vi "CALC_Phi_theta_etc_(offline).vi"(0 "Input cluster of data":T1, 1 "SB size":u8, 2 "Bridge swap":bool, 3 "Use alternative magnets orientation":bool, 4 "Twisted neck":bool) -> (5 "Animal coordinates":T2)   [LabVIEW 2018, in "Tracker.lvlib"]
uses:
  Tracker.lvlib
  Controls/CTL_Animal_Coordinates_and_Speed.ctl
  Controls/CTL_Cage_Coords.ctl
  Common_Resources.lvlib
  <vilib>/ptbypt/NI_PtbyPt.lvlib
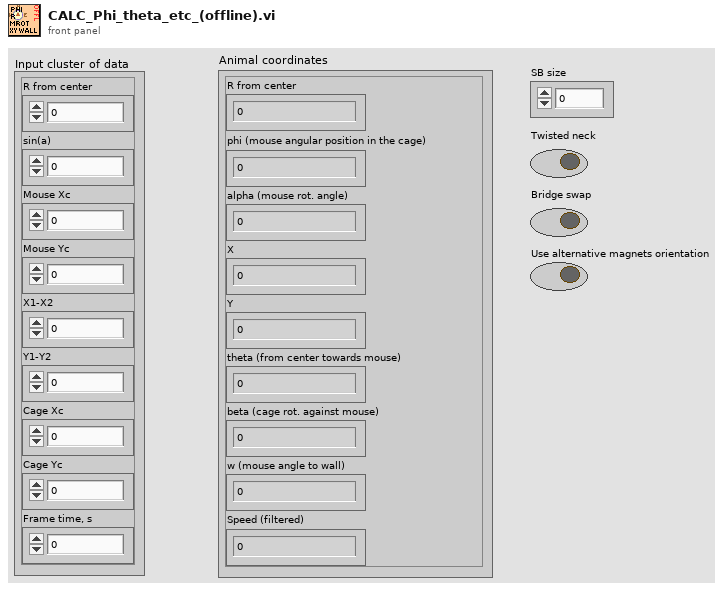
[diagram p1: front panel]
types:
  T1 = typedef "Common_Resources.lvlib/CTL_Cage_Coords.ctl" = cluster{"R from center":dbl, "sin(a)":dbl, "Mouse Xc":dbl, "Mouse Yc":dbl, "X1-X2":dbl, "Y1-Y2":dbl, "Cage Xc":dbl, "Cage Yc":dbl, "Frame time, s":dbl}
  T2 = typedef "Common_Resources.lvlib/CTL_Animal_Coordinates_and_Speed.ctl" = cluster{"R from center":dbl, "phi (mouse angular position in the cage)":dbl, "alpha (mouse rot. angle)":dbl, "X":dbl, "Y":dbl, "theta (from center towards mouse)":dbl, "beta (cage rot. against mouse)":dbl, "w (mouse angle to wall)":dbl, "Speed (filtered)":dbl}
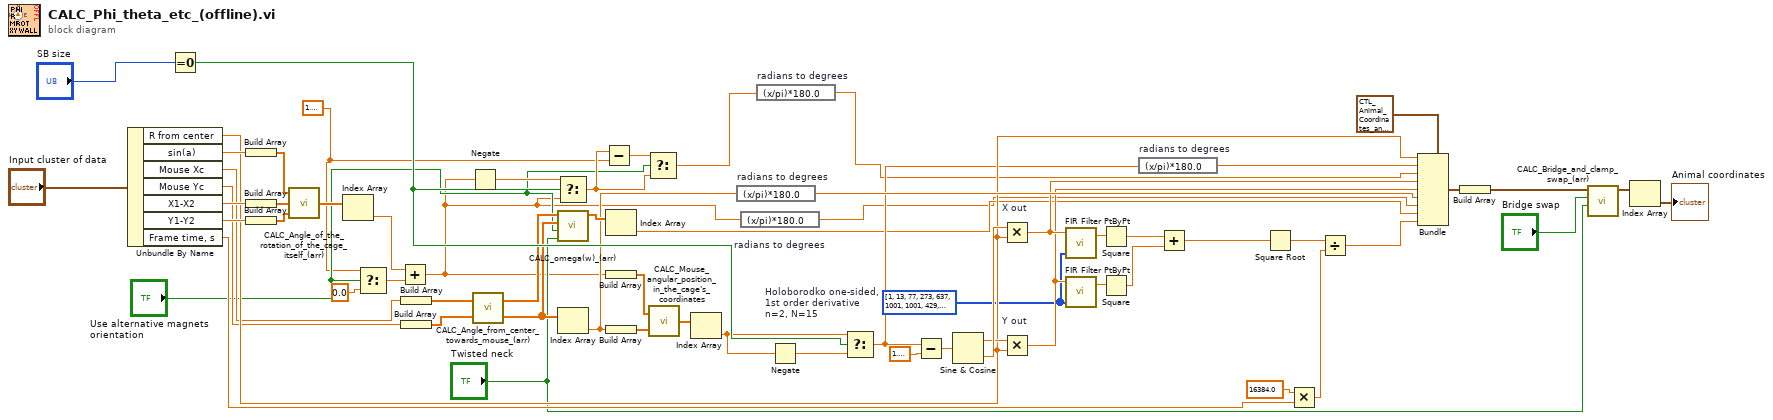
[diagram p0: block diagram]
diagram:
  w5 = 1.5707963267948966
  w36 = i32[] [1, 13, 77, 273, 637, 1001, 1001, 429, -429, -1001, -1001, -637, -273, -77, -13, -1]  # Holoborodko one-sided, 1st order derivative n=2, N=15
  n1 = Unbundle By Name("Input cluster of data") -> ("R from center"=w55:dbl, "sin(a)"=w58:dbl, "Mouse Xc"=w21:dbl, "Mouse Yc"=w20:dbl, "X1-X2"=w57:dbl, "Y1-Y2"=w56:dbl, "Frame time, s"=w30:dbl)
  n2 = Equal To 0?(x="SB size") -> (x = 0?=w39:bool)
  n3 = Build Array(w58) -> (w25:dbl[])
  n4 = Build Array(w57) -> (w24:dbl[])
  n5 = Build Array(w56) -> (w23:dbl[])
  n6 = call "CALC_Angle_of_the_rotation_of_the_cage_itself_(arr).vi"("Y1-Y2"=w23, "X1-X2"=w24, "sin(a)"=w25) -> ("Cage rot. angle, rad"=w50:dbl[])
  n7 = Index Array(array=w50) -> (element=w22:dbl)  [unwired: 1 in]
  n8 = Select(t=w5, s="Use alternative magnets orientation", f=0.0) -> (s? t:f=w48:dbl)
  n9 = Add(x=w22, y=w48) -> (x+y=w4:dbl)
  n10 = Build Array(w21) -> (w19:dbl[])
  n11 = Build Array(w20) -> (w18:dbl[])
  n12 = Negate(x=w4) -> (-x=w46:dbl)
  n13 = call "CALC_Angle_from_center_towards_mouse_(arr).vi"("Mouse Yc"=w18, "Mouse Xc"=w19) -> ("abs(theta) < pi, rad"=w11:dbl[], "theta, rad"=w12:dbl[])
  n14 = Select(t=w46, s=w39, f=w4) -> (s? t:f=w47:dbl)
  n15 = call "CALC_omega(w)_(arr).vi"("Twisted neck (F)"="Twisted neck", "Alt. magnets orientation (F)"="Use alternative magnets orientation", "abs(theta) < pi, rad"=w11, "theta, rad"=w12) -> ("w, deg"=w41:dbl[])  [unwired: 7 in]
  n16 = Index Array(array=w11) -> (element=w14:dbl)  [unwired: 1 in]
  n17 = Subtract(x=w47, y=w5) -> (x-y=w49:dbl)
  n18 = Index Array(array=w41) -> (element=w13:dbl)  [unwired: 1 in]
  n19 = Build Array(w4) -> (w15:dbl[])
  n20 = Build Array(w14) -> (w17:dbl[])
  n21 = Select(t=w49, s="Use alternative magnets orientation", f=w47) -> (s? t:f=w2:dbl)
  n22 = call "CALC_Mouse_angular_position_in_the_cage's_coordinates.vi"("abs(theta) < pi, rad"=w17, "a, rad"=w15) -> ("phi, rad"=w44:dbl[])
  n23 = Index Array(array=w44) -> (element=w16:dbl)  [unwired: 1 in]
  n24 = expression code="(x/pi)*180.0" "radians to degrees"(w14) -> (w60:dbl)
  n25 = expression code="(x/pi)*180.0" "radians to degrees"(w4) -> (w3:dbl)
  n26 = expression code="(x/pi)*180.0" "radians to degrees"(w2) -> (w1:dbl)
  n27 = Negate(x=w16) -> (-x=w43:dbl)
  n28 = Select(t=w16, s=w39, f=w43) -> (s? t:f=w45:dbl)
  n29 = Subtract(x=w45, y=1.5707963267948966) -> (x-y=w62:dbl)
  n30 = Sine & Cosine(0:w62) -> (1:w63:dbl, 2:w64:dbl)
  n31 = Multiply "X out"(x=w64, y=w55) -> (x*y=w38:dbl)
  n32 = Multiply "Y out"(x=w63, y=w55) -> (x*y=w37:dbl)
  n33 = call <vilib>:"FIR Filter PtByPt.vi"("Forward Coefficients"=w36, "x"=w38) -> ("Filtered x"=w35:dbl)  [unwired: 2 in, 1 out]
  n34 = call <vilib>:"FIR Filter PtByPt.vi"("Forward Coefficients"=w36, "x"=w37) -> ("Filtered x"=w34:dbl)  [unwired: 2 in, 1 out]
  n35 = Square(x=w35) -> (x^2=w33:dbl)
  n36 = Square(x=w34) -> (x^2=w32:dbl)
  n37 = expression code="(x/pi)*180.0" "radians to degrees"(w45) -> (w54:dbl)
  n38 = Add(x=w33, y=w32) -> (x+y=w31:dbl)
  n39 = Square Root(x=w31) -> (sqrt(x)=w27:dbl)
  n40 = Multiply(x=16384.0 ("y"), y=w30) -> (x*y=w26:dbl)
  n41 = Divide(x=w27, y=w26) -> (x/y=w29:dbl)
  n42 = Bundle(cluster=T2 {"R from center"=0.0, "phi (mouse angular position in the cage)"=0.0, "alpha (mouse rot. angle)"=0.0, "X"=0.0, "Y"=0.0, "theta (from center towards mouse)"=0.0, "beta (cage rot. against mouse)"=0.0, "w (mouse angle to wall)"=0.0, "Speed (filtered)"=0.0} ("Output data cluster 2"), "R from center"=w55, "phi (mouse angular position in the cage)"=w54, "alpha (mouse rot. angle)"=w1, "X"=w38, "Y"=w37, "theta (from center towards mouse)"=w60, "beta (cage rot. against mouse)"=w3, "w (mouse angle to wall)"=w13, "Speed (filtered)"=w29) -> (w8:T2)
  n43 = Build Array(w8) -> (w7:T2[])
  n44 = call "CALC_Bridge_and_clamp_swap_(arr).vi"("Twisted neck"="Twisted neck", "Bridge swap"="Bridge swap", "Data array in"=w7) -> ("Data array out"=w42:T2[])  [unwired: 8 in]
  n45 = Index Array(array=w42) -> (element=→"Animal coordinates":T2)  [unwired: 1 in]
